vi "Write Mulitple Strings.vi"(5 "Mulitple Strings":bool, 9 "Boolean in":refnum<class "Boolean.lvclass">) -> (3 "Boolean out":refnum<class "Boolean.lvclass">)   [LabVIEW 2014, in "Boolean.lvclass"]
uses:
  Boolean.lvclass
  Boolean.lvclass/Boolean.ctl
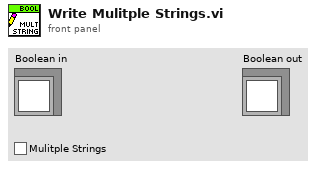
[diagram p1: front panel]
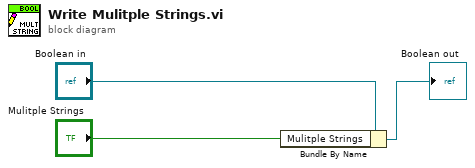
[diagram p0: block diagram]
diagram:
  n1 = Bundle By Name(cluster="Boolean in", "Mulitple Strings"="Mulitple Strings") -> (→"Boolean out":refnum<class "Boolean.lvclass">)
